vi "Trio - Get Program List.vi"(1 "Controller Directory":string, 2 "Exclusion List":string[](array[string])) -> (0 "Programs List":string[](array[string]))   [LabVIEW 2020, in "TrioMotion Controller.lvlib"]
uses:
  TrioMotion Controller.lvlib
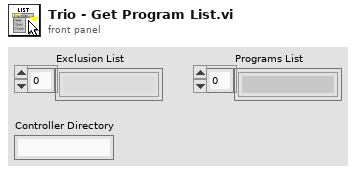
[diagram p1: front panel]
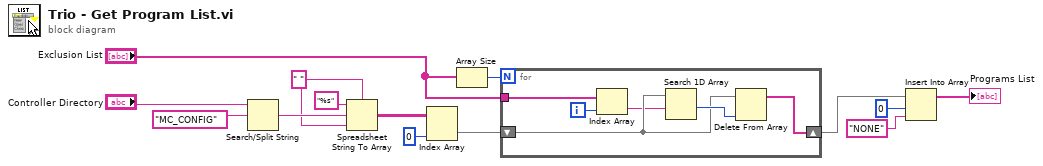
[diagram p0: block diagram]
diagram:
  w7 = " " ("delimiter (Tab)")
  n1 = Search/Split String(string="Controller Directory", search string/char (-)="MC_CONFIG") -> (match + rest of string=w8:string)  [unwired: 1 in, 2 out]
  n2 = Spreadsheet String To Array(delimiter (Tab)=w7, format string="%s", spreadsheet string=w8, array type (2D Dbl)=w7) -> (array=w4:string[][])
  n3 = Index Array(array=w4, index (col)=0 ("disabled index (col)")) -> (element=w10:string[])  [unwired: 1 in]
  n4 = Array Size(array="Exclusion List") -> (size(s)=w1:i32)
  n5 = for {
    N: w1 -> [_]
    tunnel: "Exclusion List" -> [w17]
    shift-right: [w15] -> w11
    shift-left: w10 -> [w18]
    i -> [w19]
    n6 = Index Array(array=w17, index=w19) -> (element=w16:string)
    n7 = Search 1D Array(1D array=w18, element=w16) -> (index of element=w20:i32)  [unwired: 1 in]
    n8 = Delete From Array(array=w18, index=w20) -> (array with subset deleted=w15:string[])  [unwired: 1 in, 1 out]
  }
  n9 = Insert Into Array(array=w11, index=0, new element="NONE") -> (→"Programs List":string[])
